vi "Get Commit Hash.vi"(10 "Commit ID":i32, 11 "Peer Review":refnum<class "Peer Review.lvclass">) -> (3 "Hash":string)   [LabVIEW 2020, in "Peer Review.lvclass"]
uses:
  Peer Review.lvclass
  Peer Review.lvclass/Peer Review.ctl
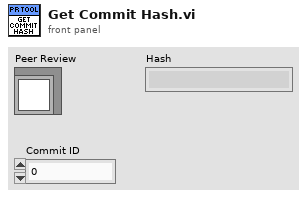
[diagram p1: front panel]
types:
  T1 = typedef "Peer Review.lvclass/Commit Info.ctl" = cluster{"Commit ID":i32, "Hash":string, "Merge Commit?":bool, "Merge Hash":string, "Author":string, "Time Stamp":timestamp, "Description":string, "File Count":i32, "File List":string[]}
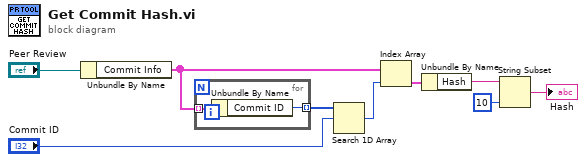
[diagram p0: block diagram]
diagram:
  n1 = Unbundle By Name("Peer Review") -> ("Commit Info"=w4:T1[])
  n2 = for {
    tunnel: w4 -> [w11] mode=indexing
    tunnel: [w10] -> w2 mode=indexing
    n3 = Unbundle By Name(w11) -> ("Commit ID"=w10:i32)
  }
  n4 = Search 1D Array(1D array=w2, element="Commit ID") -> (index of element=w5:i32)  [unwired: 1 in]
  n5 = Index Array(array=w4, index=w5) -> (element=w6:T1)
  n6 = Unbundle By Name(w6) -> ("Hash"=w7:string)
  n7 = String Subset(string=w7, length (rest)=10 ("length (rest)")) -> (substring=→"Hash":string)  [unwired: 1 in]
